vi "DC Motor Controller SCADA.vi"() -> ()   [LabVIEW 2015]
uses:
  <vilib>/Instr/_visa.llb/VISA Configure Serial Port (Instr).vi
  <vilib>/picture/3D Picture Control/Object/Create Object (name).vi
  <vilib>/picture/3D Picture Control/NI_3D Picture Control.lvlib
panel:
  out "Motor Postion":refnum<vi>(3d-picture)
  in  "Reset Positon Display":bool
  in  "STOP":bool
  out "?":dbl
  out "?":dbl
  in  "flow control (0:none)":u16(ring) items=["None", "XON/XOFF", "RTS/CTS", "XON/XOFF & RTS/CTS", "DTR/DSR", "XON/XOFF & DTR/DSR"]
  out "Connection Status":bool
  in  "termination char\n(0xA = '\\n' = LF)":u8=10 format="%.0x"
  in  "Enable Termination\nChar (T)":bool=TRUE
  in  "stop bits (10: 1 bit)":u16(ring)=10 items=["1.0"=10, "1.5"=15, "2.0"=20]
  in  "parity (0:none)":enum16{"None", "Odd", "Even", "Mark", "Space"}(ring)
  in  "data bits (8)":u16=8 min=5 max=8 step=1
  in  "Baud Rate":u32=9600
  out "?":dbl
  in  "Get PID Parameters":bool
  in  "Apply PID \nSettings":bool
  in  "Set Motor":bool
  in  "Motor Position":dbl
  in  "KD - Input":dbl
  in  "KI - Input":dbl
  in  "KP - Input":dbl
  in  "Controller Port":refnum<visa-resource-name>
  in  "Connect":bool
  # "Communication"
  # "PID Controller"
  # "Motor Postion Control"
  # "Motor Target Postion:"
  # "MCU KP"
  # "MCU KI"
  # "MCU KD"
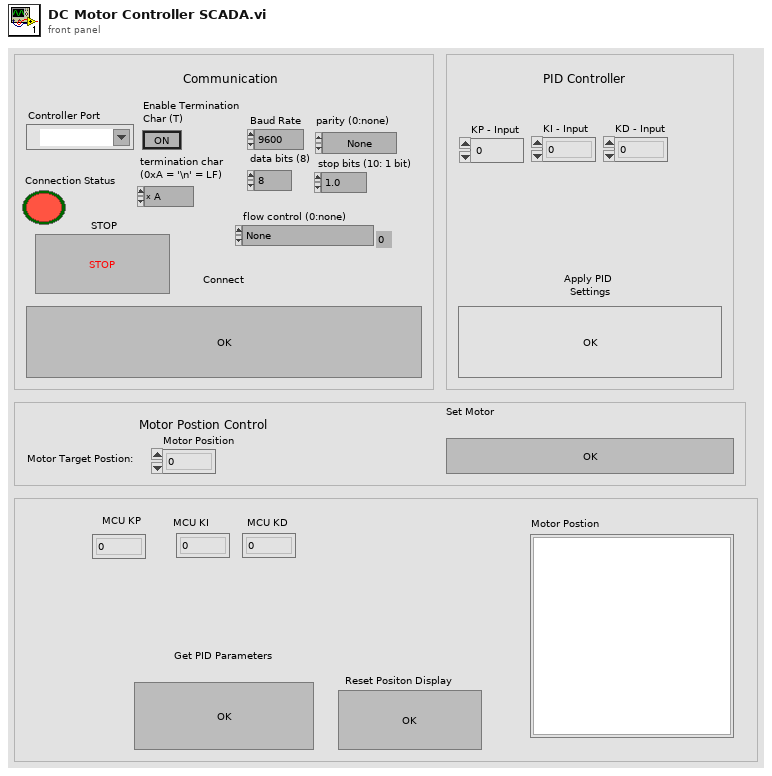
[diagram p1: front panel]
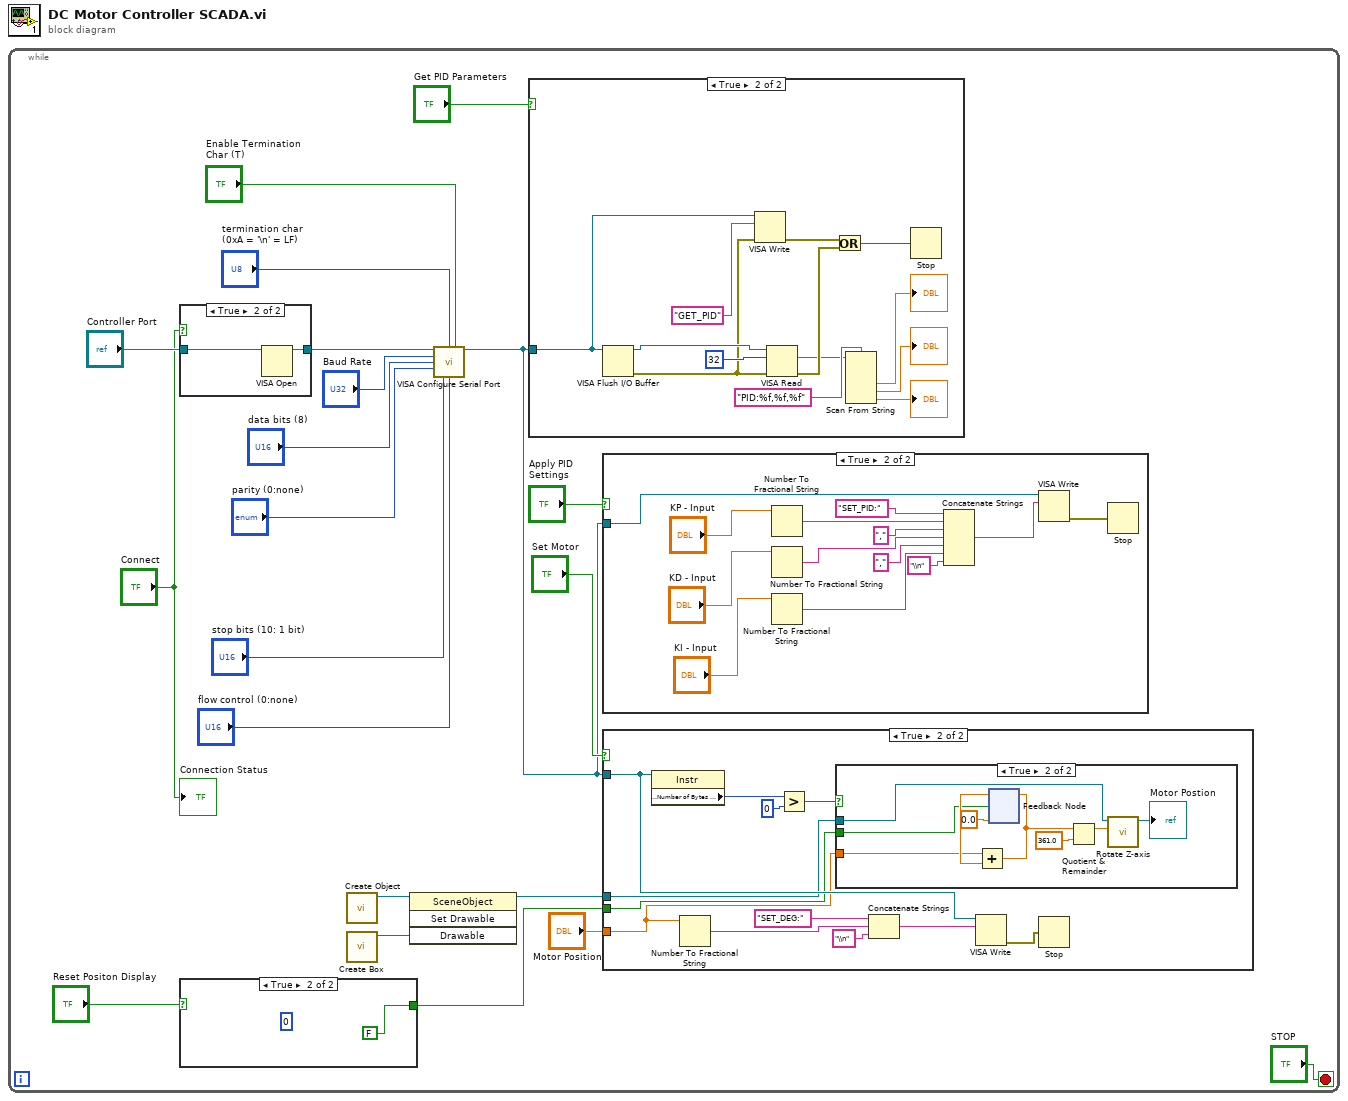
[diagram p0: block diagram]
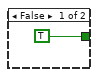
[diagram p2: hidden frame]
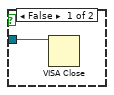
[diagram p3: hidden frame]
diagram:
  n1 = while {
    stop <- "STOP" stop-if-true
    n2 = case shown="True" "Connect" {
      tunnel: [_ w26] -> w17
      tunnel: "Controller Port" -> [w24 w25]
      frame False {
        n3 = VISA Close(VISA resource name=w24) -> ()  [unwired: 1 in, 1 out]
      }
      frame True {
        n4 = VISA Open(VISA resource name=w25) -> (VISA resource name=w26:refnum<visa-resource-name>)  [unwired: 4 in, 1 out]
      }
    }
    n5 = case shown="True" "Reset Positon Display" {
      tunnel: [TRUE FALSE] -> w5
      frame False {
      }
      frame True {
        (unwired) 0
      }
    }
    n6 = call-poly <vilib>:"Create Object.vi"() -> ("Scene:New Object"=w3:refnum<vi>)  [unwired: 10 in, 1 out]
    n7 = call <vilib>:"Create Box.vi"() -> ("New Box Refnum"=w4:refnum<vi>)  [unwired: 10 in, 1 out]
    n8 = invoke class="SceneObject" method="Set Drawable"(reference=w3, "Drawable"=w4) -> (reference out=w2:refnum<vi>)  [unwired: 2 in, 3 out]
    n9 = call-poly "VISA Configure Serial Port"("VISA resource name"=w17, "termination char\n(0xA = '\\n' = LF)"="termination char\n(0xA = '\\n' = LF)", "Enable Termination\nChar (T)"="Enable Termination\nChar (T)", "baud rate (9600)"="Baud Rate", "data bits (8)"="data bits (8)", "parity (0:none)"="parity (0:none)", "stop bits (10: 1 bit)"="stop bits (10: 1 bit)", "flow control (0:none)"="flow control (0:none)") -> ("VISA resource name out"=w16:refnum<visa-resource-name>)  [unwired: 6 in, 1 out]
    n10 = case shown="True" "Get PID Parameters" {
      tunnel: w16 -> [_ w36]
      frame False {
      }
      frame True {
        n11 = VISA Flush I/O Buffer(VISA resource name=w36) -> (VISA resource name out=w39:refnum<visa-resource-name>, error out=w33:errorcluster)  [unwired: 2 in]
        n12 = VISA Write(VISA resource name=w36, write buffer="GET_PID", error in (no error)=w33) -> (error out=w32:errorcluster)  [unwired: 2 out]
        n13 = VISA Read(VISA resource name=w39, byte count=u32 32, error in (no error)=w33) -> (read buffer=w27:string, error out=w31:errorcluster)  [unwired: 2 out]
        n14 = Or(x=w32, y=w31) -> (x .or. y?=w30:bool)
        n15 = Scan From String(format string="PID:%f,%f,%f", input string=w27) -> (output 1=→"?":dbl, output 2=→"?":dbl, output 3=→"?":dbl)  [unwired: 5 in, 3 out]
        n16 = Stop(stop? (T)=w30) -> ()
      }
    }
    n17 = case shown="True" "Apply PID \nSettings" {
      tunnel: w16 -> [_ w68]
      frame False {
      }
      frame True {
        n18 = Number To Fractional String(number="KP - Input") -> (F-format string=w67:string)  [unwired: 3 in]
        n19 = Number To Fractional String(number="KD - Input") -> (F-format string=w66:string)  [unwired: 3 in]
        n20 = Number To Fractional String(number="KI - Input") -> (F-format string=w65:string)  [unwired: 3 in]
        n21 = Concatenate Strings("SET_PID:", w67, ",", w66, ",", w65, "\\n") -> (w69:string)
        n22 = VISA Write(VISA resource name=w68, write buffer=w69) -> (error out=w61:errorcluster)  [unwired: 1 in, 2 out]
        n23 = Stop(stop? (T)=w61) -> ()
      }
    }
    n24 = case shown="True" "Set Motor" {
      tunnel: w16 -> [_ w44]
      tunnel: w5 -> [_ w42]
      tunnel: "Motor Position" -> [_ w41]
      tunnel: w2 -> [_ w40]
      frame False {
      }
      frame True {
        n25 = property class="Instr"(reference=w44) -> ("Serial Settings:Number of Bytes at Serial Port"=w47:u32)  [unwired: 1 in, 2 out]
        n26 = Number To Fractional String(number=w41) -> (F-format string=w48:string)  [unwired: 3 in]
        n27 = Greater?(x=w47, y=u32 0) -> (0:w46:bool)
        n28 = case shown="True" w46 {
          tunnel: w42 -> [_ w56]
          tunnel: w41 -> [_ w55]
          tunnel: w40 -> [_ w54]
          frame False {
          }
          frame True {
            n29 = feedback #1(0.0) -> (w58:dbl)
            n30 = Add(x=w55, y=w58) -> (x+y=w59:dbl)
            n31 = feedback-in #1(w59, w56) -> ()
            n32 = Quotient & Remainder(x=w59, y=361.0) -> (x-y*floor(x/y)=w53:dbl)  [unwired: 1 out]
            n33 = call <vilib>:"Rotate Z-axis.vi"("angle"=w53, "Scene Object In"=w54) -> ("Scene Object Out"=→"Motor Postion":refnum<vi>)  [unwired: 8 in, 1 out]
          }
        }
        n34 = Concatenate Strings("SET_DEG:", w48, "\\n") -> (w51:string)
        n35 = VISA Write(VISA resource name=w44, write buffer=w51) -> (error out=w43:errorcluster)  [unwired: 1 in, 2 out]
        n36 = Stop(stop? (T)=w43) -> ()
      }
    }
    "Connection Status" <- "Connect"
  }
